vi "写入IO编译.vi"(10 "维数大小":i32=2, 11 "Write Data":bool[](array[boolean])) -> (3 "数据":u32[](array[numeric]))   [LabVIEW 2014]
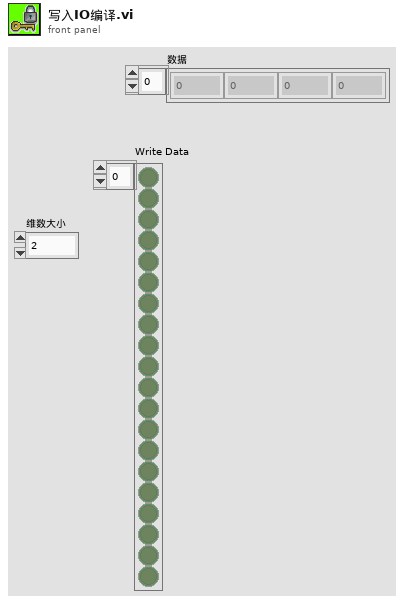
[diagram p1: front panel]
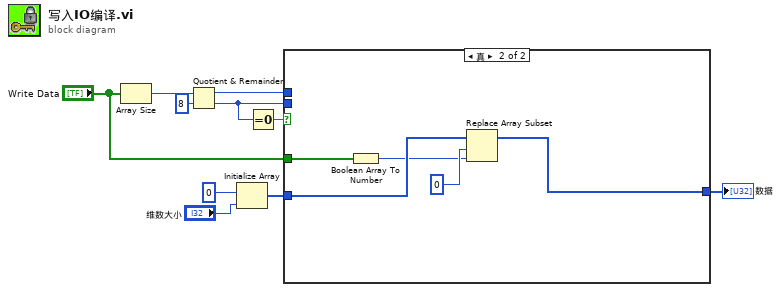
[diagram p0: block diagram]
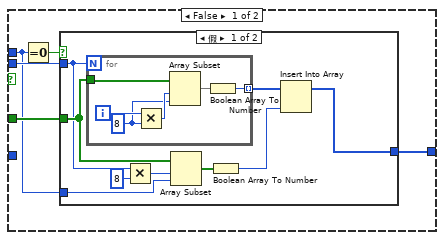
[diagram p2: hidden frame]
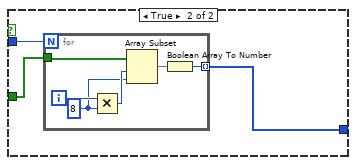
[diagram p3: hidden frame]
diagram:
  n1 = Array Size(array="Write Data") -> (size(s)=w9:i32)
  n2 = Quotient & Remainder(x=w9, y=8) -> (x-y*floor(x/y)=w6:i32, floor(x/y)=w7:i32)
  n3 = Initialize Array(0, "维数大小") -> (w4:i32[])
  n4 = Equal To 0?(x=w7) -> (x = 0?=w5:bool)
  n5 = case shown="真" w5 {
    tunnel: "Write Data" -> [w13 w44]
    tunnel: w4 -> [_ w43]
    tunnel: [w12 w40] -> w1
    tunnel: w7 -> [w14 _]
    tunnel: w6 -> [w11 _]
    frame False {
      n6 = Equal To 0?(x=w11) -> (x = 0?=w15:bool)
      n7 = case shown="假" w15 {
        tunnel: w14 -> [w21 w33]
        tunnel: w13 -> [w23 w32]
        tunnel: [w16 w31] -> w12
        tunnel: w11 -> [w19 _]
        frame False {
          n8 = for {
            N: w21 -> [_]
            tunnel: w23 -> [w30]
            tunnel: [w25] -> w24 mode=indexing
            i -> [w29]
            w27 = 8 ("y")
            n9 = Multiply(x=w29, y=w27) -> (x*y=w28:i32)
            n10 = Array Subset(array=w30, index=w28, length=w27) -> (w26:bool[])
            n11 = Boolean Array To Number(Boolean array=w26) -> (number=w25:u32)
          }
          n12 = Multiply(x=w21, y=8) -> (x*y=w20:i32)
          n13 = Array Subset(array=w23, index=w20, length=w19) -> (w18:bool[])
          n14 = Boolean Array To Number(Boolean array=w18) -> (number=w17:u32)
          n15 = Insert Into Array(array=w24, new element=w17) -> (w16:u32[])  [unwired: 1 in]
        }
        frame True {
          n16 = for {
            N: w33 -> [_]
            tunnel: w32 -> [w39]
            tunnel: [w34] -> w31 mode=indexing
            i -> [w38]
            w36 = 8 ("y")
            n17 = Multiply(x=w38, y=w36) -> (x*y=w37:i32)
            n18 = Array Subset(array=w39, index=w37, length=w36) -> (w35:bool[])
            n19 = Boolean Array To Number(Boolean array=w35) -> (number=w34:u32)
          }
        }
      }
    }
    frame True {
      n20 = Boolean Array To Number(Boolean array=w44) -> (number=w41:u32)
      n21 = Replace Array Subset(array=w43, new element=w41, index=0 ("索引 (行)")) -> (w40:i32[])
    }
  }
  "数据" <- w1
